vi "isDefaultStyle.vi"(8 "error in (no error)":errorcluster, 11 "Style in":refnum<class "Style.lvclass">) -> (0 "error out":errorcluster, 2 "isDefault":bool, 3 "Style out":refnum<class "Style.lvclass">)   [LabVIEW 2020, in "Styles.lvlib" / "Style.lvclass"]
uses:
  Style.lvclass
  Get Default Style.vi
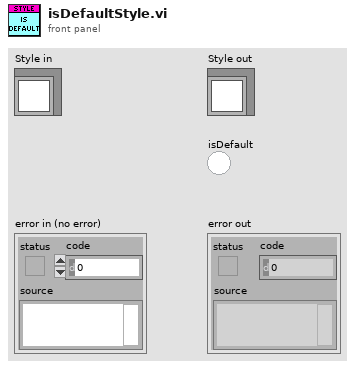
[diagram p1: front panel]
types:
  T1 = typedef "Styles.lvlib/Underline--ring.ctl" = i32
  T2 = typedef "Styles.lvlib/Alignment--ring.ctl" = i32
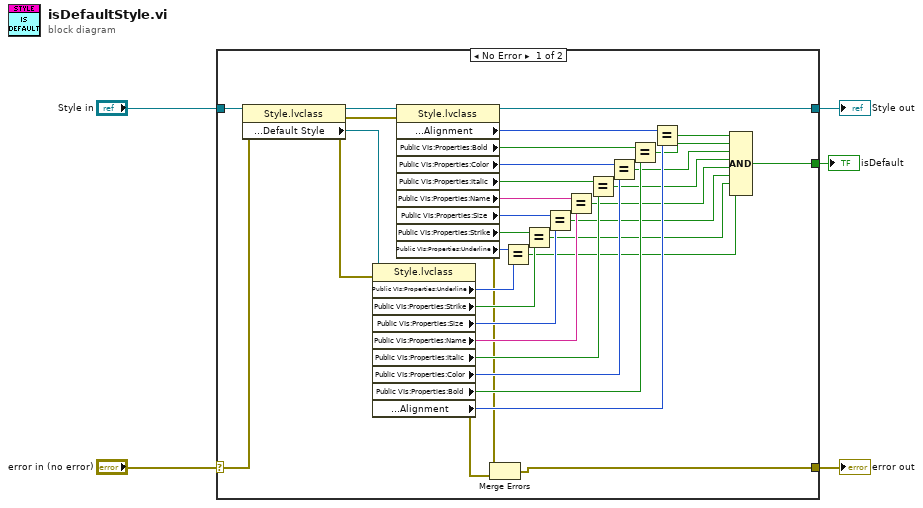
[diagram p0: block diagram]
diagram:
  n1 = case shown="No Error" "error in (no error)" {
    selector: "error in (no error)" -> [w10 w41]
    tunnel: [w7 w41] -> w4
    tunnel: [w36 w40] -> w2
    tunnel: "Style in" -> [w39 w40]
    tunnel: [w11 _] -> w1
    frame No Error {
      n2 = property class="Style.lvclass"(reference=w39, error in=w10) -> (reference out=w37:refnum<class "Style.lvclass">, error out=w9:errorcluster, "Public VIs:Properties:Default Style"=w38:refnum<class "Style.lvclass">)
      n3 = property class="Style.lvclass"(reference=w38, error in=w9) -> (error out=w6:errorcluster, "Public VIs:Properties:Underline"=w34:T1, "Public VIs:Properties:Strike"=w32:bool, "Public VIs:Properties:Size"=w30:i32, "Public VIs:Properties:Name"=w28:string, "Public VIs:Properties:Italic"=w26:bool, "Public VIs:Properties:Color"=w24:u32, "Public VIs:Properties:Bold"=w21:bool, "Public VIs:Properties:Alignment"=w20:T2)  [unwired: 1 out]
      n4 = property class="Style.lvclass"(reference=w37, error in=w9) -> (reference out=w36:refnum<class "Style.lvclass">, error out=w8:errorcluster, "Public VIs:Properties:Alignment"=w22:T2, "Public VIs:Properties:Bold"=w23:bool, "Public VIs:Properties:Color"=w25:u32, "Public VIs:Properties:Italic"=w27:bool, "Public VIs:Properties:Name"=w29:string, "Public VIs:Properties:Size"=w31:i32, "Public VIs:Properties:Strike"=w33:bool, "Public VIs:Properties:Underline"=w35:T1)
      n5 = Merge Errors(w8, w6) -> (w7:errorcluster)
      n6 = Equal?(x=w35, y=w34) -> (x = y?=w12:bool)
      n7 = Equal?(x=w33, y=w32) -> (x = y?=w13:bool)
      n8 = Equal?(x=w31, y=w30) -> (x = y?=w14:bool)
      n9 = Equal?(x=w29, y=w28) -> (x = y?=w15:bool)
      n10 = Equal?(x=w27, y=w26) -> (x = y?=w16:bool)
      n11 = Equal?(x=w25, y=w24) -> (x = y?=w17:bool)
      n12 = Equal?(x=w23, y=w21) -> (x = y?=w18:bool)
      n13 = Equal?(x=w22, y=w20) -> (x = y?=w19:bool)
      n14 = Compound Arithmetic op=AND(w19, w18, w17, w16, w15, w14, w13, w12) -> (w11:bool)
    }
    frame Error {
    }
  }
  "error out" <- w4
  "Style out" <- w2
  "isDefault" <- w1
